vi "RPM Sensor(SubVI).vi"() -> (1 "Edge":bool, 2 "RPM Max 1":dbl, 4 "RPM Min 1":dbl)   [LabVIEW 2017]
uses:
  <vilib>/functionblocks/Edge Detection/Edge Detect/Edge Detect.vi
  <vilib>/functionblocks/FB Core/FB Core.xnode
  <vilib>/functionblocks/NI_FunctionBlock Libraries.lvlib
panel:
  out "Waveform Chart":dbl(graph)
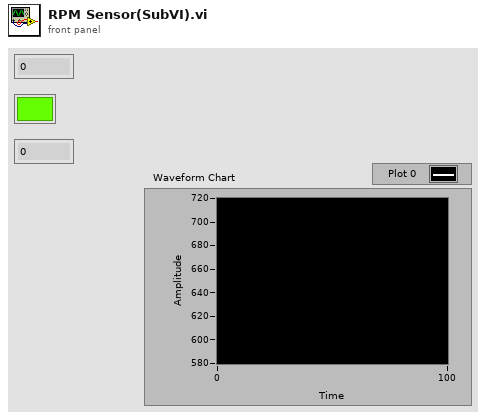
[diagram p1: front panel]
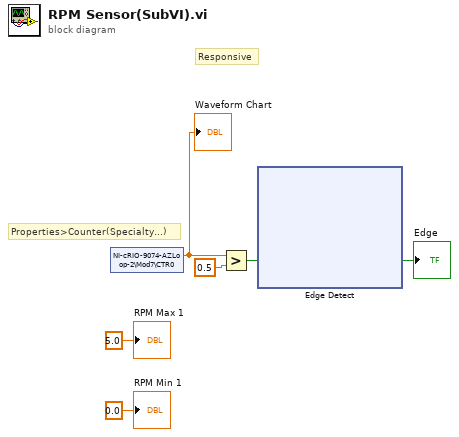
[diagram p0: block diagram]
diagram:
  # "Responsive"
  # "Properties>Counter(Specialty...)"
  n1 = shared-variable "NI-cRIO-9074-AZLoop-2\\Mod7\\CTR0"() -> (w1:dbl)  [unwired: 1 in, 1 out]
  "Waveform Chart" <- w1
  n2 = Greater?(x=w1, y=0.5) -> (0:w5:bool)
  n3 = xnode "Edge Detect"("input 2"=w5) -> ("output"=→"Edge":bool)  [unwired: 2 in, 1 out]
  "RPM Min 1" <- 0.0
  "RPM Max 1" <- 5.0
